vi "Access Platform DB Path.vi"(11 "名称或相对路径":string="database1.mdb") -> (2 "Connection information":string, 3 "Path out":string)   [LabVIEW 2016, in "Access Lib.lvlib"]
uses:
  Access Lib.lvlib
  <vilib>/Utility/sysdir.llb/System Directory Type.ctl
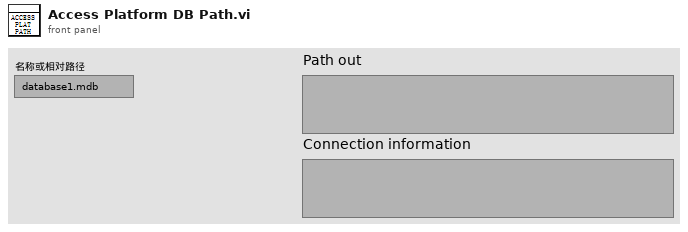
[diagram p1: front panel]
types:
  T1 = typedef "System Directory Type.ctl" = i32
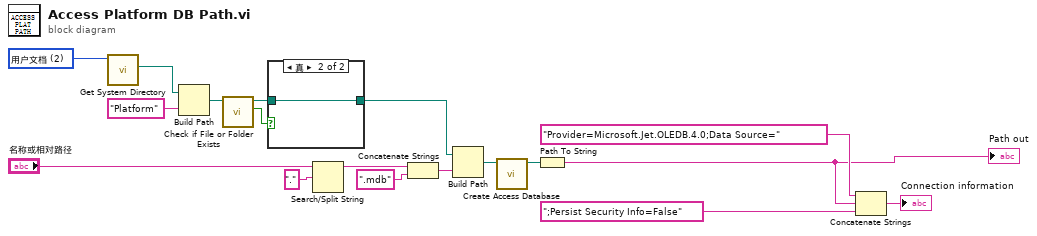
[diagram p0: block diagram]
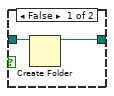
[diagram p2: hidden frame]
diagram:
  w15 = T1 2 items=["用户目录"=0, "用户桌面"=1, "用户文档"=2, "用户应用程序数据"=3, "用户设置"=4, "用户临时目录"=5, "公共文档"=6, "公共应用程序数据"=7, "公共设置"=8, "公共缓存"=13, "系统核心库"=9, "系统安装库"=10, "应用程序文件"=11, "启动盘根目录"=12] ("system directory type")
  n1 = call <vilib>:"Get System Directory.vi"("system directory type"=w15) -> ("system directory"=w14:path)  [unwired: 10 in]
  n2 = Build Path(base path=w14, name or relative path="Platform" ("名称或相对路径")) -> (appended path=w12:path)
  n3 = call <vilib>:"Check if File or Folder Exists.vi"("path"=w12) -> ("file or folder exists?"=w18:bool, "dup path"=w17:path)  [unwired: 8 in, 1 out]
  n4 = case shown="真" w18 {
    tunnel: w17 -> [w20 w21]
    tunnel: [w19 w21] -> w16
    frame False {
      n5 = Create Folder(path (use dialog)=w20) -> (created path=w19:path)  [unwired: 2 in, 2 out]
    }
    frame True {
    }
  }
  n6 = Search/Split String(string="名称或相对路径", search string/char (-)="." ("搜索字符串/字符(-)")) -> (substring before match=w10:string)  [unwired: 1 in, 2 out]
  n7 = Concatenate Strings(w10, ".mdb" ("字符串")) -> (w6:string)
  n8 = Build Path(base path=w16, name or relative path=w6) -> (appended path=w11:path)
  n9 = call "Create Access Database.vi"("路径"=w11) -> ("路径 out"=w3:path)  [unwired: 9 in, 1 out]
  n10 = Path To String(path=w3) -> (string=w2:string)
  "Path out" <- w2
  n11 = Concatenate Strings("Provider=Microsoft.Jet.OLEDB.4.0;Data Source=" ("condition"), w2, ";Persist Security Info=False" ("condition")) -> (→"Connection information":string)
